vi "Database Recordset Get Value From Field.vi"(8 "error in (no error)":errorcluster caption="错误输入（无错误）", 9 "Index":i32, 11 "Database Recordset 输入":refnum<class "Database Recordset.lvclass"> caption="DNL_LabVIEW Object in") -> (0 "error out":errorcluster caption="错误输出", 1 "Value":variant, 3 "Database Recordset 输出":refnum<class "Database Recordset.lvclass"> caption="DNL_LabVIEW Object out")   [LabVIEW 2011, in "Database Recordset.lvclass"]
uses:
  Database Recordset.lvclass
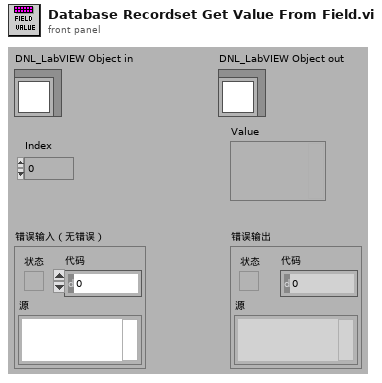
[diagram p1: front panel]
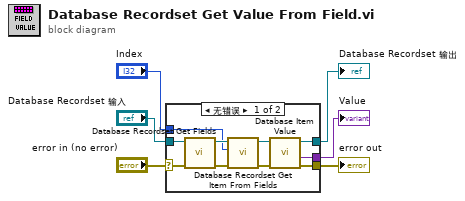
[diagram p0: block diagram]
diagram:
  n1 = case shown="无错误" "error in (no error)" {
    selector: "error in (no error)" -> [w10 w18]
    tunnel: [w7 w18] -> w5
    tunnel: [w15 w17] -> w3
    tunnel: "Database Recordset 输入" -> [w16 w17]
    tunnel: [w12 _] -> w2
    tunnel: "Index" -> [w11 _]
    frame No Error {
      n2 = call "Database Recordset Get Fields.vi"("error in (no error)"=w10, "Database Recordset 输入"=w16) -> ("error out"=w9:errorcluster, "Database Recordset 输出"=w14:refnum<class "Database Recordset.lvclass">)  [unwired: 8 in]
      n3 = call "Database Recordset Get Item From Fields.vi"("error in (no error)"=w9, "Index"=w11, "Database Recordset 输入"=w14) -> ("error out"=w8:errorcluster, "Database Recordset 输出"=w13:refnum<class "Database Recordset.lvclass">)  [unwired: 6 in, 1 out]
      n4 = call "Database Item Value.vi"("error in (no error)"=w8, "Database Recordset 输入"=w13) -> ("error out"=w7:errorcluster, "Value"=w12:variant, "Database Recordset 输出"=w15:refnum<class "Database Recordset.lvclass">)  [unwired: 7 in]
    }
    frame Error {
    }
  }
  "error out" <- w5
  "Database Recordset 输出" <- w3
  "Value" <- w2
